vi "timing test.vi"() -> ()   [LabVIEW 2018]
panel:
  out "return type":i32
  out "Indices":u32[](array[numeric])
  out "Array":dbl[](array[numeric])
  in  "Test count":i32=20
  in  "Sample length":i32=20
  in  "SV length":i32=20
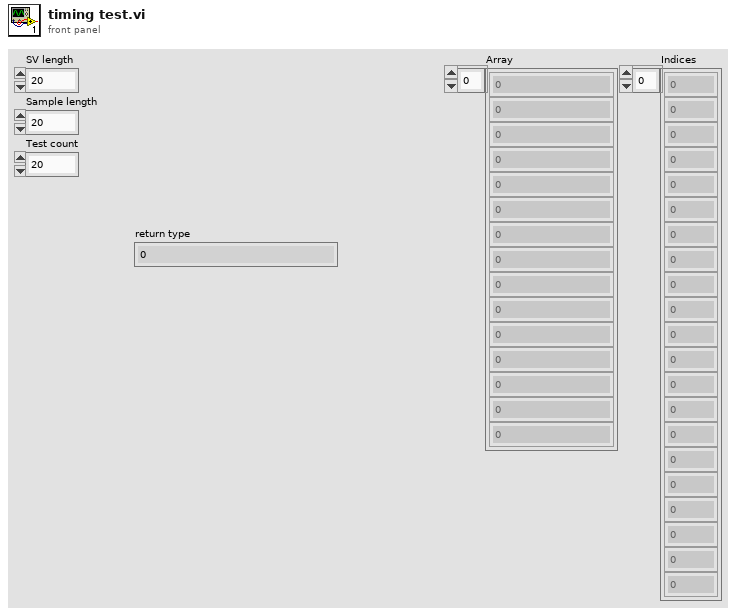
[diagram p1: front panel]
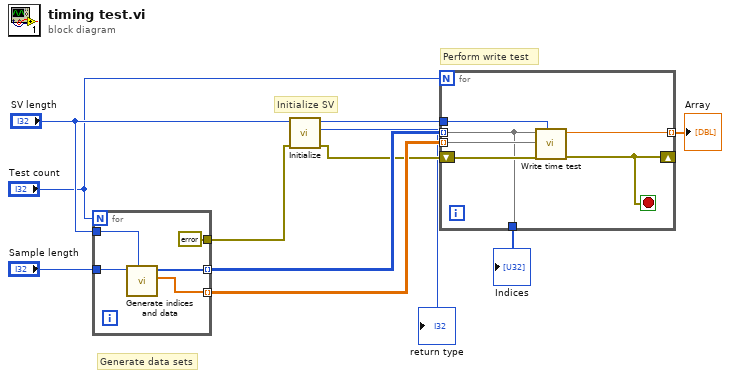
[diagram p0: block diagram]
diagram:
  # "Perform write test"
  # "Generate data sets"
  # "Initialize SV"
  n1 = for {
    N: "Test count" -> [_]
    tunnel: "Sample length" -> [w16]
    tunnel: "SV length" -> [w15]
    tunnel: [w14] -> w7 mode=indexing
    tunnel: [w13] -> w6 mode=indexing
    tunnel: [errorcluster {"status"=FALSE, "code"=0, "source"=""} ("Error In")] -> w2
    n2 = call "Generate indices and data.vi"("Length"=w15, "Sample size"=w16) -> ("Data"=w13:dbl[], "Indices"=w14:u32[])  [unwired: 8 in]
  }
  n3 = call "Initialize.vi"("Error In"=w2, "Size"="SV length") -> ("Error Out"=w5:errorcluster, "return type"=→"return type":i32, "Map id"=w8:i32)  [unwired: 7 in]
  n4 = for {
    N: "Test count" -> [_]
    tunnel: w8 -> [w20]
    tunnel: w7 -> [w17] mode=indexing
    tunnel: w6 -> [w21] mode=indexing
    shift-right: [w18] -> _
    shift-left: w5 -> [w22]
    tunnel: [w19] -> w4 mode=indexing
    tunnel: [w17] -> w3
    stop <- w18 stop-if-true
    n5 = call "Write time test.vi"("Map id"=w20, "Error In"=w22, "Data"=w21, "Indices"=w17) -> ("Error Out"=w18:errorcluster, "dt"=w19:dbl)  [unwired: 6 in]
  }
  "Array" <- w4
  "Indices" <- w3
